vi "Write Signal Suffix.vi"(8 "error in (no error)":errorcluster, 10 "Signal Suffix":string, 11 "IMD_ACP in":refnum<class "IMD_ACP.lvclass">) -> (0 "error out":errorcluster, 3 "IMD_ACP out":refnum<class "IMD_ACP.lvclass">)   [LabVIEW 2018, in "SeqAuto Evaluations.lvlib" / "IMD_ACP.lvclass"]
uses:
  IMD_ACP.lvclass
  IMD_ACP.lvclass/IMD_ACP.ctl
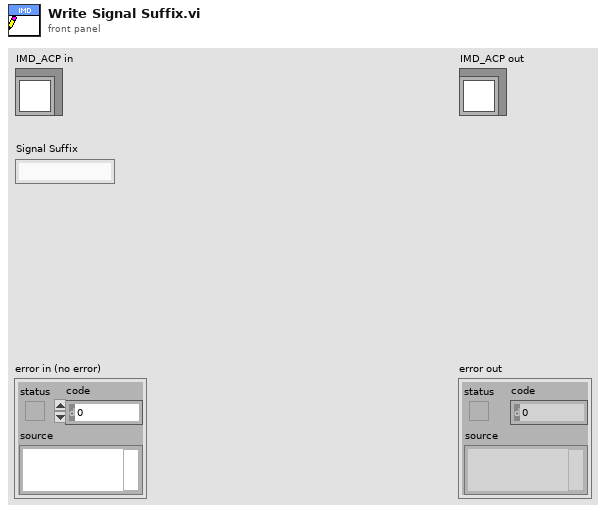
[diagram p1: front panel]
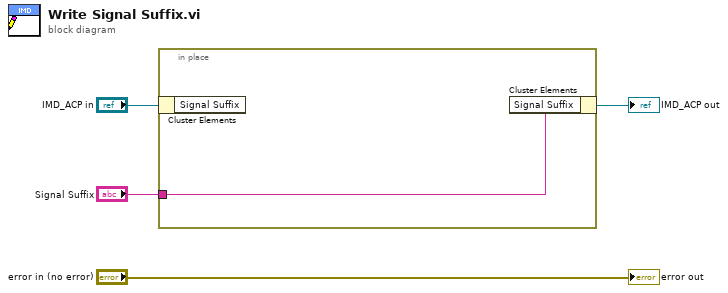
[diagram p0: block diagram]
diagram:
  n1 = in-place {
    in-place-border: "Signal Suffix" -> [w5]
    n2 = in-place-cluster #1("IMD_ACP in") -> ()  [unwired: 1 out]
    n3 = in-place-cluster #1("Signal Suffix"=w5) -> (→"IMD_ACP out":refnum<class "IMD_ACP.lvclass">)
  }
  "error out" <- "error in (no error)"
